vi "wiskunde.vi"() -> ()   [LabVIEW 2014]
uses:
  Kimematics Param.ctl
  <vilib>/myRIO/Common/Instrument Driver Framework/myRIO v1.0/PWM/vis/myRIO v1.1 Open PWM.vi
  <vilib>/myRIO/Common/Instrument Driver Framework/myRIO v1.0/UART/vis/myRIO v1.0 Close UART.vi
  <vilib>/myRIO/Common/Instrument Driver Framework/Utilities/vis/Validate Channels.vi
  <vilib>/myRIO/Common/Instrument Driver Framework/myRIO v1.0/PWM/vis/myRIO v1.0 Reserve PWM.vi
  <vilib>/myRIO/Common/Instrument Driver Framework/myRIO v1.0/PWM/vis/myRIO v1.0 Build MUX Configuration PWM.vi
  <vilib>/myRIO/Common/Instrument Driver Framework/myRIO v1.0/Resource Manager/vis/myRIO v1.0 Reserve Channel List.vi
  <vilib>/myRIO/Common/Instrument Driver Framework/myRIO v1.0/Resource Manager/vis/myRIO v1.0 Create Configuration List.vi
  <vilib>/myRIO/Common/Instrument Driver Framework/myRIO v1.0/Resource Manager/vis/myRIO v1.0 Reserve Channel.vi
  <vilib>/myRIO/Common/Instrument Driver Framework/myRIO v1.0/Resource Manager/vis/myRIO v1.0 Unreserve Channel.vi
  <vilib>/myRIO/Common/Instrument Driver Framework/myRIO v1.0/Resource Manager/vis/myRIO v1.0 Build Mutex Name.vi
  <vilib>/Utility/VariantDataType/GetNumericInfo.vi
  <vilib>/Utility/error.llb/Error Cluster From Error Code.vi
  <vilib>/myRIO/Common/Instrument Driver Framework/myRIO v1.0/myRIO v1.1 Open.vi
  <vilib>/myRIO/Common/Instrument Driver Framework/Utilities/vis/IO Manager.vi
  <vilib>/myRIO/Common/Instrument Driver Framework/Utilities/vis/Configuration Manager.vi
  <vilib>/myRIO/Common/Instrument Driver Framework/myRIO v1.0/Resource Manager/vis/myRIO v1.0 Configure IO.vi
  <vilib>/myRIO/Common/Instrument Driver Framework/myRIO v1.0/myRIO v1.0 Close.vi
  <vilib>/myRIO/Common/Instrument Driver Framework/myRIO v1.0/PWM/vis/myRIO v1.0 Write PWM.vi
  <vilib>/myRIO/Common/Instrument Driver Framework/Utilities/vis/FPGA Ref Manager.vi
  <vilib>/myRIO/Common/Instrument Driver Framework/myRIO v1.0/myRIO v1.0 Reset FPGA.vi
  <vilib>/myRIO/Common/Instrument Driver Framework/myRIO v1.0/IRQ/vis/myRIO v1.0 IRQ Info FGV.vi
  <vilib>/myRIO/Common/Instrument Driver Framework/myRIO v1.0/IRQ/vis/myRIO v1.0 Timer IRQ Info FGV.vi
  <vilib>/myRIO/Common/Instrument Driver Framework/myRIO v1.0/IRQ/vis/myRIO v1.0 ISR Agent.vi
  <vilib>/myRIO/Instrument Drivers/Onboard IO/PWM/PWM.lvlib
  <vilib>/myRIO/Instrument Drivers/Utilities/Utilities.lvlib
panel:
  in  "[ESC]":bool
  in  "Z":dbl(slide) scale=10.0..40.0
  in  "Y":dbl(slide) scale=-20.0..20.0
  in  "X":dbl(slide) scale=-20.0..20.0
  out "element 3":dbl
  out "element 2":dbl
  out "element":dbl
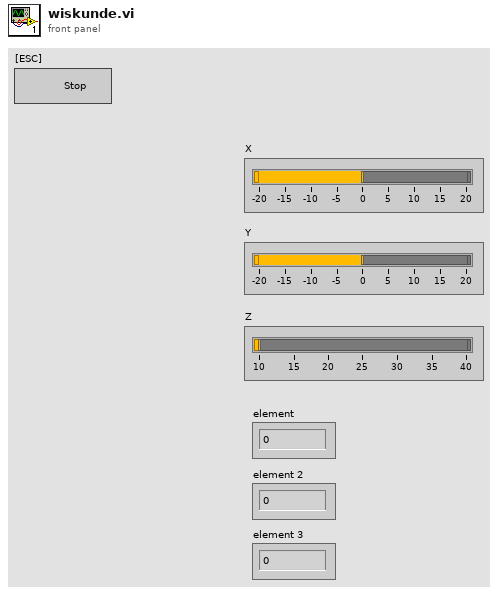
[diagram p1: front panel]
types:
  T1 = typedef "Kimematics Param.ctl" = cluster{"Length of arms \"a\" (cm)":dbl, "Length of arms \"b\" (cm)":dbl, "Length of  base \"r\" (cm)":dbl, "Length of platform \"h\" (cm)":dbl, "Phi (deg)":dbl[], "Upper limit of Theta":dbl, "Lower limit of Theta":dbl}
  T2 = typedef "PWM.lvlib/PWM Reference.ctl" = cluster{"myRIO Reference":T3, "PWM Channels Enum":T7, "PWM Configuration":T8}
  T3 = typedef "myRIO Generic Hardware Reference.ctl" = cluster{"myRIO Model":T4, "myRIO Hardware Reference":T5}
  T4 = typedef "Hardware Version Enum.ctl" = enum16{"Unknown", "myRIO-1900", "myRIO-1950"}
  T5 = typedef "myRIO v1.0 Reference.ctl" = cluster{"Generic FPGA Reference":T6, "Allow multiple opens":bool}
  T6 = typedef "Generic FPGA Reference.ctl" = refnum<k20>
  T7 = typedef "PWM Channels Enum.ctl" = enum16{"Not Connected", "C/PWM0", "C/PWM1", "A/PWM0", "A/PWM1", "A/PWM2", "B/PWM0", "B/PWM1", "B/PWM2"}
  T8 = typedef "PWM.lvlib/PWM Configuration.ctl" = cluster{"Frequency":dbl, "Duty Cycle":dbl}
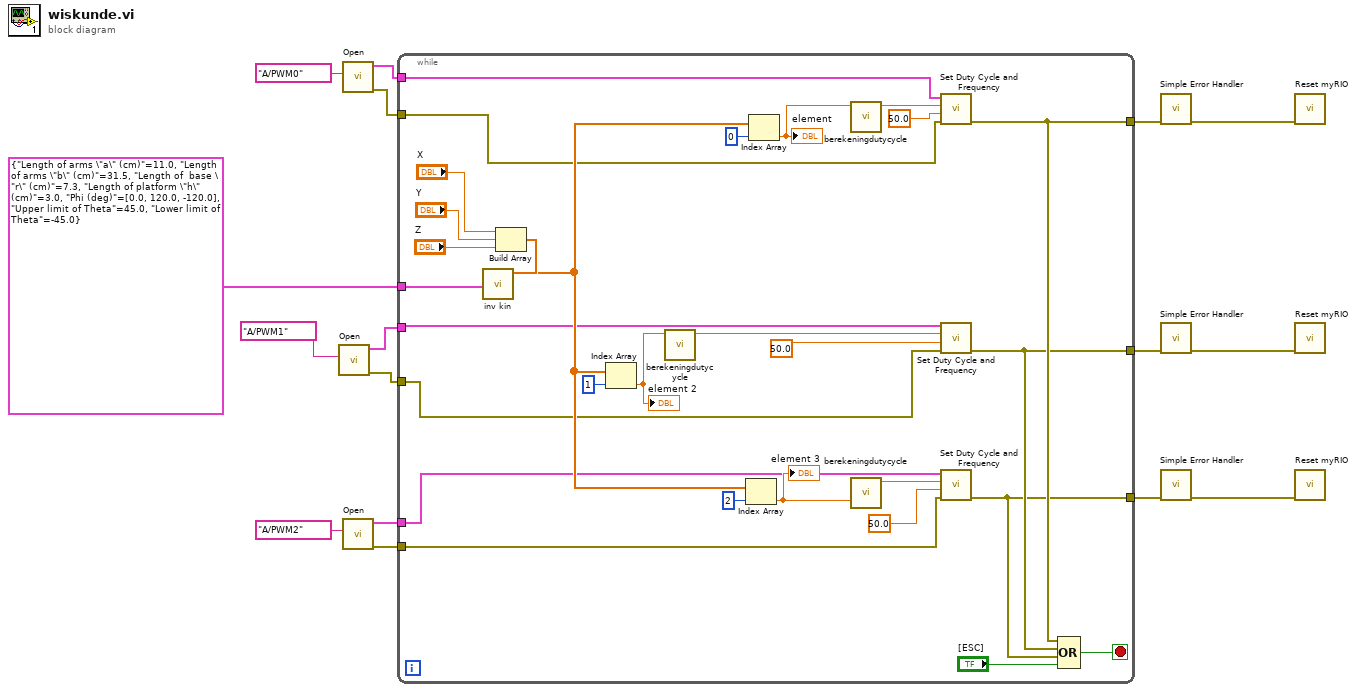
[diagram p0: block diagram]
diagram:
  n1 = call <vilib>:"Open.vi"("Channel Name"=tag "A/PWM1") -> ("error out"=w4:errorcluster, "PWM Ref Out"=w5:T2)  [unwired: 9 in]
  n2 = call <vilib>:"Open.vi"("Channel Name"=tag "A/PWM0") -> ("error out"=w6:errorcluster, "PWM Ref Out"=w7:T2)  [unwired: 9 in]
  n3 = call <vilib>:"Open.vi"("Channel Name"=tag "A/PWM2") -> ("error out"=w2:errorcluster, "PWM Ref Out"=w3:T2)  [unwired: 9 in]
  n4 = while {
    tunnel: [w20] -> w16
    tunnel: [w21] -> w15
    tunnel: [w22] -> w14
    tunnel: w7 -> [w28]
    tunnel: w6 -> [w17]
    tunnel: w5 -> [w27]
    tunnel: w4 -> [w24]
    tunnel: w3 -> [w26]
    tunnel: w2 -> [w25]
    tunnel: T1 {"Length of arms \"a\" (cm)"=11.0, "Length of arms \"b\" (cm)"=31.5, "Length of  base \"r\" (cm)"=7.3, "Length of platform \"h\" (cm)"=3.0, "Phi (deg)"=[0.0, 120.0, -120.0], "Upper limit of Theta"=45.0, "Lower limit of Theta"=-45.0} ("Kinematics Param") -> [w23]
    stop <- w18 stop-if-true
    n5 = Build Array("X", "Y", "Z") -> (w45:dbl[])
    n6 = call "inv kin.vi"("Kinematics Param"=w23, "Point of TCF (X,Y,Z)"=w45) -> ("Theta (deg)"=w41:dbl[])  [unwired: 7 in, 2 out]
    n7 = Index Array(array=w41, index=1) -> (element=w32:dbl)
    "element 2" <- w32
    n8 = call "berekeningdutycycle.vi"("Graden"=w32) -> ("Numeric"=w29:dbl)  [unwired: 10 in]
    n9 = Index Array(array=w41, index=2) -> (element=w31:dbl)
    "element 3" <- w31
    n10 = Index Array(array=w41, index=0) -> (element=w34:dbl)
    "element" <- w34
    n11 = call "berekeningdutycycle.vi"("Graden"=w34) -> ("Numeric"=w33:dbl)  [unwired: 10 in]
    n12 = call "berekeningdutycycle.vi"("Graden"=w31) -> ("Numeric"=w30:dbl)  [unwired: 10 in]
    n13 = call <vilib>:"Set Duty Cycle and Frequency.vi"("error in (no error)"=w17, "Frequency [Hz]"=50.0, "Duty Cycle"=w33, "PWM Ref In"=w28) -> ("error out"=w22:errorcluster)  [unwired: 5 in, 1 out]
    n14 = call <vilib>:"Set Duty Cycle and Frequency.vi"("error in (no error)"=w24, "Frequency [Hz]"=50.0, "Duty Cycle"=w29, "PWM Ref In"=w27) -> ("error out"=w21:errorcluster)  [unwired: 5 in, 1 out]
    n15 = call <vilib>:"Set Duty Cycle and Frequency.vi"("error in (no error)"=w25, "Frequency [Hz]"=50.0, "Duty Cycle"=w30, "PWM Ref In"=w26) -> ("error out"=w20:errorcluster)  [unwired: 5 in, 1 out]
    n16 = Compound Arithmetic op=OR(w22, w21, w20, "[ESC]") -> (w18:bool)
  }
  n17 = call <vilib>:"Simple Error Handler.vi"("error in (no error)"=w14) -> ("error out"=w11:errorcluster)  [unwired: 4 in, 4 out]
  n18 = call <vilib>:"Simple Error Handler.vi"("error in (no error)"=w15) -> ("error out"=w12:errorcluster)  [unwired: 4 in, 4 out]
  n19 = call <vilib>:"Simple Error Handler.vi"("error in (no error)"=w16) -> ("error out"=w13:errorcluster)  [unwired: 4 in, 4 out]
  n20 = call <vilib>:"Reset myRIO.vi"("error in (no error)"=w11) -> ()  [unwired: 10 in, 1 out]
  n21 = call <vilib>:"Reset myRIO.vi"("error in (no error)"=w12) -> ()  [unwired: 10 in, 1 out]
  n22 = call <vilib>:"Reset myRIO.vi"("error in (no error)"=w13) -> ()  [unwired: 10 in, 1 out]
